vi "Configure Game.vi"(0 "input cluster":refnum<class "Game.lvclass">, 1 "This VI":refnum<vi>, 2 "Shield":refnum<vi>, 3 "SCORE":refnum<vi>, 5 "error in (no error)":errorcluster, 6 "STAR":refnum<vi>, 7 "Background":refnum<vi>, 8 "Score":refnum<vi>, 9 "Grapes":refnum<vi>, 10 "Board Game":refnum<vi>, 11 "Image Ring":refnum<vi>) -> (14 "Application out":refnum<class "Game.lvclass">, 19 "error out":errorcluster)   [LabVIEW 2021, in "Game.lvclass"]
uses:
  Game.lvclass
  Backgroud_v2.ctl
  GameEl_class/private/Enum Direction.ctl
  Snake_class/Snake.lvclass
  Fruit_class/Fruit.lvclass
  Shield/Shield.lvclass
  Grape/Grape.lvclass
  Mouse/Mouse.lvclass
  Cricket/Cricket.lvclass
  Star/Star.lvclass
  Imposible_Snake_v2/LVApp/Modules/Sound Manager/Typedefs/Sound Effects.ctl
  Game.lvclass/Game.ctl
  Star/Star.lvclass/Star.ctl
  Bomb/Bomb.lvclass
  Grape/Grape.lvclass/Grape.ctl
  Board Game_class/Board Game.lvclass/Board Game.ctl
  <vilib>/numeric/Random Number (Range) DBL.vi
  Board Game_class/Board Game.lvclass
  GameEl_class/GameEl.lvclass
  Imposible_Snake_v2/LVApp/Modules/Sound Manager/Sound Manager.lvlib
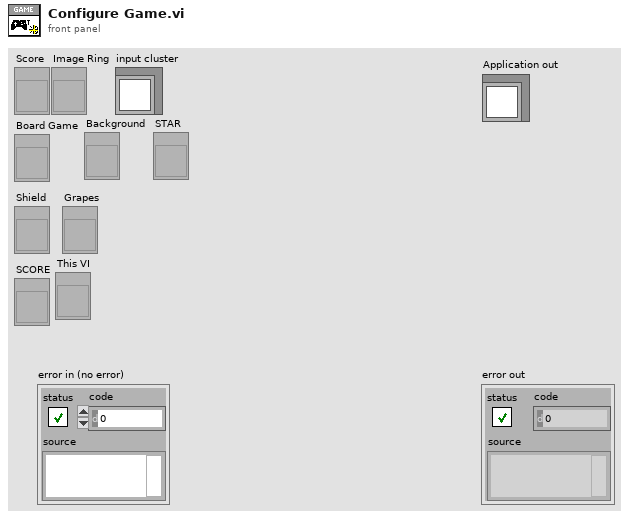
[diagram p1: front panel]
types:
  T1 = typedef "Sound Manager.lvlib/Sound Effects.ctl" = enum16{"Bomb In", "Bomb Out", "Bomb Touched", "Game Over", "Victory", "Eat", "10 Fruits", "Eat2", "Eat3", "Eat4", "MaxShield", "Shield", "10p", "Grape In", "Grape Out", "20p", "30p", "40p", "50p", "60p", "70p", "80p", "90p", "100p", "All shields cracked", "Mouse In", "Mouse Out", "Mouse Eaten", "Grape Eaten", "States Recover", "Broken Shield", "Bonus", "Happy Time", "explode", "Game over musica", "Back Music", "Shield Catch", "Evil lough", "Cricket In", "Cricket eaten", "Lets Go", "Jump1", "Jump2", "Jump3", "Unstoppable", "Troll Music", "winner", "menu"}
  T2 = typedef "GameEl.lvclass/Enum Direction.ctl" = enum16{"Up", "Down", "Forward", "Backward"}
  T3 = cluster{"millisecond timer value":u32, "Elapsed":u32}
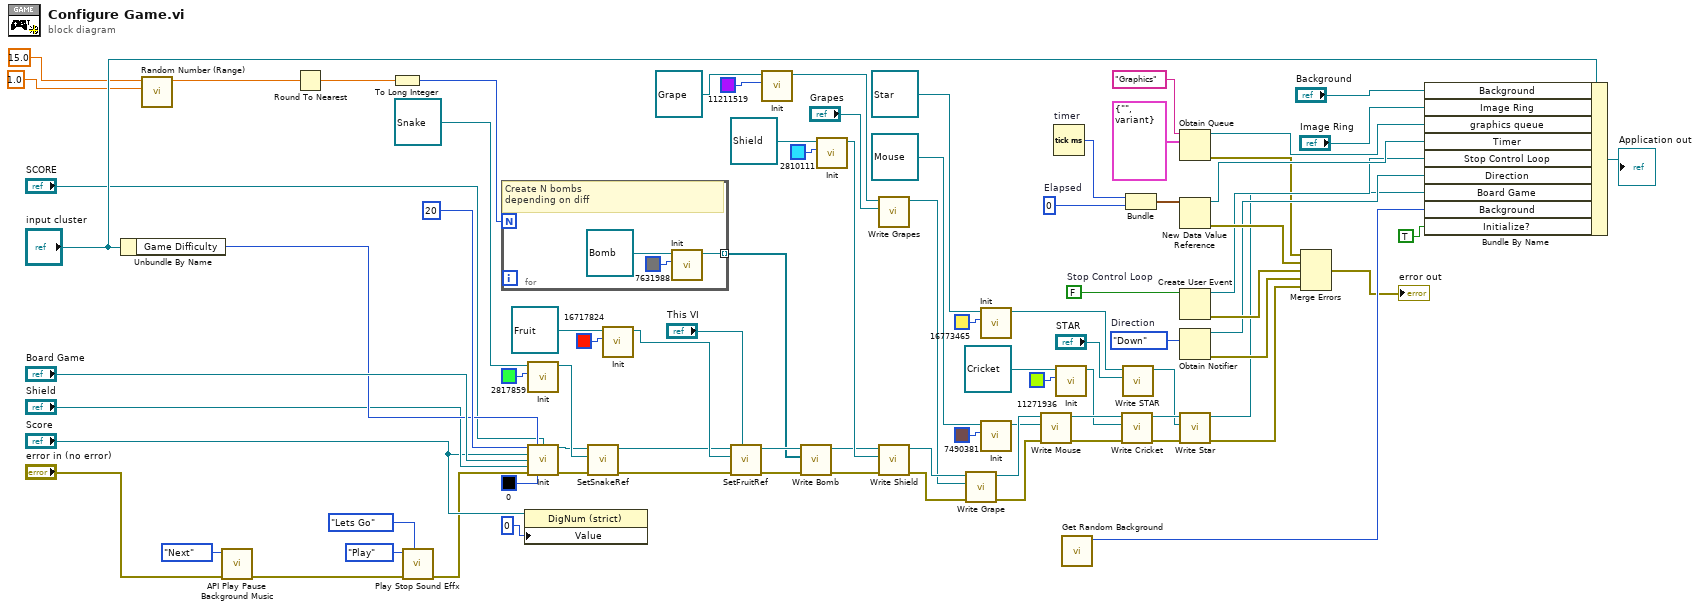
[diagram p0: block diagram]
diagram:
  w26 = u32 0  # Elapsed
  w76 = FALSE  # Stop Control Loop
  w82 = Enum_Direction."Down"  # Direction
  n1 = Unbundle By Name("input cluster") -> ("Game Difficulty"=w65:u32)
  n2 = call-poly <vilib>:"Random Number (Range).vi"("lower bound (0)"=1.0 ("Low"), "upper bound (100)"=15.0 ("High")) -> ("number"=w32:dbl)  [unwired: 9 in]
  n3 = call "API Play Pause Background Music.vi"("Error In"="error in (no error)", "Function"=enum16{"Pause", "Resume", "Next"}."Next") -> ("error in (no error)"=w4:errorcluster)  [unwired: 9 in]
  n4 = Round To Nearest(number=w32) -> (nearest integer value=w31:dbl)
  n5 = To Long Integer(number=w31) -> (32bit integer=w28:i32)
  n6 = call "Play Stop Sound Effx.vi"("Sound Effect"=Sound_Effects."Lets Go", "Error In"=w4, "Function"=enum16{"Play", "Stop"}."Play") -> ("error in (no error)"=w1:errorcluster)  [unwired: 8 in]
  n7 = for {
    N: w28 -> [_]
    tunnel: [w89] -> w64 mode=indexing
    # "Create N bombs\ndepending on diff"
    n8 = call-dynamic "Init.vi"("Colour"=u32 7631988, "GameEl in"=refnum<class "Bomb.lvclass"> refnum ("Bomb In")) -> ("GameEl out"=w89:refnum<class "Bomb.lvclass">)  [unwired: 8 in, 1 out]
  }
  n9 = property class="DigNum (strict)"(reference="Score", "Value"=u16 0) -> ()  [unwired: 1 in, 2 out]
  n10 = call-dynamic "Init.vi"("Colour"=u32 2817859, "Snake In"=refnum<class "Snake.lvclass"> refnum) -> ("object out"=w83:refnum<class "Snake.lvclass">)  [unwired: 8 in, 1 out]
  n11 = call "Init.vi"("Size"=u16 20, "Game Difficulty Out"=w65, "SCORE"="SCORE", "Score"="Score", "Board Game"="Board Game", "Shield"="Shield", "error in (no error)"=w1, "Colour"=u32 0) -> ("Board Game out"=w77:refnum<class "Board Game.lvclass">, "error out"=w80:errorcluster)  [unwired: 6 in]
  n12 = call-dynamic "SetSnakeRef.vi"("Error In"=w80, "SnakeRef"=w83, "object in"=w77) -> ("Error Out"=w79:errorcluster, "object out"=w78:refnum<class "Board Game.lvclass">)  [unwired: 7 in]
  n13 = call-dynamic "Init.vi"("Colour"=u32 16717824, "GameEl in"=refnum<class "Fruit.lvclass"> refnum ("Object in")) -> ("GameEl out"=w81:refnum<class "Fruit.lvclass">)  [unwired: 8 in, 1 out]
  n14 = call-dynamic "SetFruitRef.vi"("This VI"="This VI", "Error In"=w79, "FruitRef"=w81, "object in"=w78) -> ("Error Out"=w69:errorcluster, "object out"=w70:refnum<class "Board Game.lvclass">)  [unwired: 6 in]
  n15 = call-dynamic "Init.vi"("Colour"=u32 11211519, "GameEl in"=refnum<class "Grape.lvclass"> refnum ("Grape.lvclass")) -> ("GameEl out"=w44:refnum<class "Grape.lvclass">)  [unwired: 8 in, 1 out]
  n16 = call "Write Bomb.vi"("error in (no error)"=w69, "Array"=w64, "Board Game in"=w70) -> ("error out"=w55:errorcluster, "Board Game out"=w57:refnum<class "Board Game.lvclass">)  [unwired: 7 in]
  n17 = call-dynamic "Init.vi"("Colour"=u32 2810111, "GameEl in"=refnum<class "Shield.lvclass"> refnum ("Shield in")) -> ("GameEl out"=w58:refnum<class "Shield.lvclass">)  [unwired: 8 in, 1 out]
  n18 = call "Write Grapes.vi"("Grapes"="Grapes", "Grape in"=w44) -> ("Grape out"=w43:refnum<class "Grape.lvclass">)  [unwired: 8 in, 1 out]
  n19 = call "Write Shield.vi"("error in (no error)"=w55, "Shield.lvclass"=w58, "Board Game in"=w57) -> ("error out"=w45:errorcluster, "Board Game out"=w56:refnum<class "Board Game.lvclass">)  [unwired: 7 in]
  n20 = call "Write Grape.vi"("error in (no error)"=w45, "Grape.lvclass"=w43, "Board Game in"=w56) -> ("error out"=w40:errorcluster, "Board Game out"=w46:refnum<class "Board Game.lvclass">)  [unwired: 7 in]
  n21 = call-dynamic "Init.vi"("Colour"=u32 16773465, "GameEl in"=refnum<class "Star.lvclass"> refnum ("Star.lvclass")) -> ("GameEl out"=w12:refnum<class "Star.lvclass">)  [unwired: 8 in, 1 out]
  n22 = call-dynamic "Init.vi"("Colour"=u32 7490381, "GameEl in"=refnum<class "Mouse.lvclass"> refnum ("Mouse.lvclass")) -> ("GameEl out"=w37:refnum<class "Mouse.lvclass">)  [unwired: 8 in, 1 out]
  n23 = call "Write Mouse.vi"("error in (no error)"=w40, "Mouse.lvclass"=w37, "Board Game in"=w46) -> ("error out"=w39:errorcluster, "Board Game out"=w22:refnum<class "Board Game.lvclass">)  [unwired: 7 in]
  n24 = Tick Count (ms) "timer"() -> (millisecond timer value=w71:u32)
  n25 = call-dynamic "Init.vi"("Colour"=u32 11271936, "GameEl in"=refnum<class "Cricket.lvclass"> refnum ("Cricket.lvclass")) -> ("GameEl out"=w21:refnum<class "Cricket.lvclass">)  [unwired: 8 in, 1 out]
  n26 = call "Get Random Background.vi"() -> ("Numeric"=w29:u16)  [unwired: 11 in]
  n27 = call "Write Cricket.vi"("error in (no error)"=w39, "Cricket.lvclass"=w21, "Board Game in"=w22) -> ("error out"=w23:errorcluster, "Board Game out"=w14:refnum<class "Board Game.lvclass">)  [unwired: 7 in]
  n28 = call "Write STAR.vi"("STAR"="STAR", "Star in"=w12) -> ("Star out"=w10:refnum<class "Star.lvclass">)  [unwired: 8 in, 1 out]
  n29 = Bundle("millisecond timer value"=w71, "Elapsed"=w26) -> (w27:T3)  [unwired: 1 in]
  n30 = Obtain Queue(name (unnamed)="Graphics", element data type=cluster{"Message":string, "Data":variant} {"Message"="", "Data"=variant}) -> (queue out=w62:refnum<queue>, error out=w41:errorcluster)  [unwired: 3 in, 1 out]
  n31 = New Data Value Reference(data value=w27) -> (data value reference=w61:refnum<data-value>, error out=w72:errorcluster)  [unwired: 1 in]
  n32 = Create User Event(user event datatype=w76) -> (user event=w60:refnum<user-event>, error out=w75:errorcluster)  [unwired: 1 in]
  n33 = Obtain Notifier(notification data type=w82) -> (notifier out=w59:refnum<notifier>, error out=w74:errorcluster)  [unwired: 3 in, 1 out]
  n34 = call "Write Star.vi"("error in (no error)"=w23, "Star.lvclass"=w10, "Board Game in"=w14) -> ("error out"=w15:errorcluster, "Board Game out"=w13:refnum<class "Board Game.lvclass">)  [unwired: 7 in]
  n35 = Merge Errors(w41, w72, w75, w74, w15) -> (→"error out":errorcluster)
  n36 = Bundle By Name(cluster="input cluster", "Background"="Background", "Image Ring"="Image Ring", "graphics queue"=w62, "Timer"=w61, "Stop Control Loop"=w60, "Direction"=w59, "Board Game"=w13, "Background"=w29, "Initialize?"=TRUE) -> (→"Application out":refnum<class "Game.lvclass">)
